vi "Calculate X Y Step Size.vi"(6 "Overlap Options":T3 {"Percent Overlap" max=50}, 7 "Scan Pattern":T1(ring), 8 "Error In":errorcluster, 10 "Y Axis":T2, 11 "X Axis":T2) -> (0 "Error Out":errorcluster, 1 "Array":cluster{"X":dbl, "Y":dbl}[](array[cluster]), 2 "Y Axis Out":T2, 3 "X Axis Out":T2, 4 "size(s)":i32, 5 "# X tiles":i32)   [LabVIEW 2018]
uses:
  Controls/FGV Actions.ctl
panel:
  out "XY Graph":cluster{"X":dbl, "Y":dbl}[](graph)
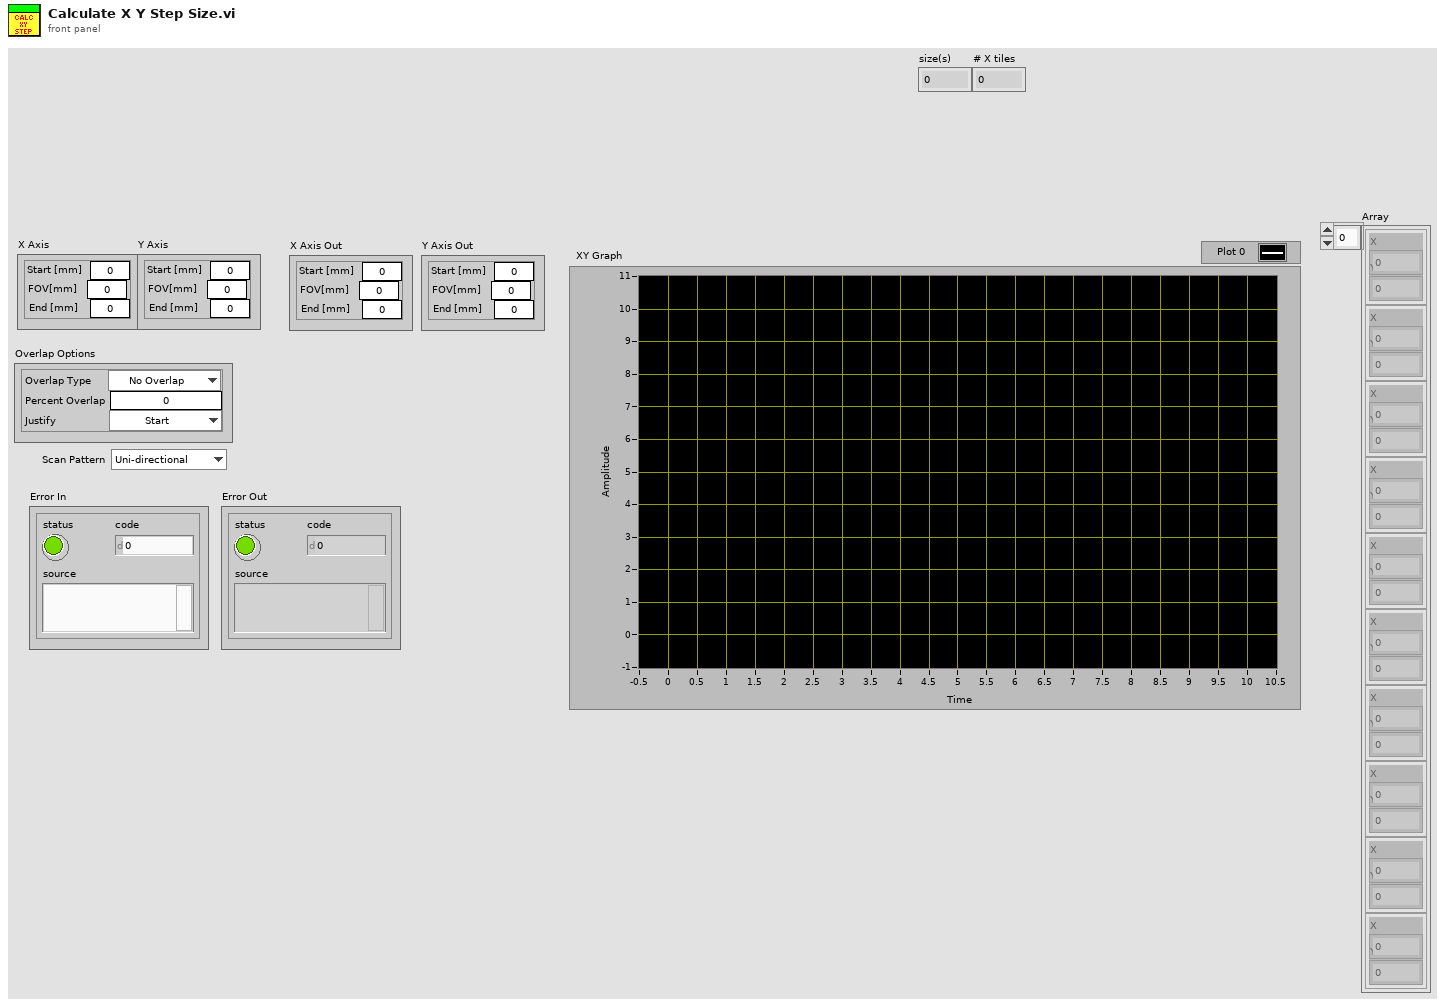
[diagram p1: front panel]
types:
  T1 = enum16{"Uni-directional", "Bi-Directional", "Spiral Out", "Spiral In"}
  T2 = cluster{"Start [mm]":dbl, "FOV[mm]":dbl, "End [mm]":dbl}
  T3 = cluster{"Overlap Type":enum16{"No Overlap", "X Only", "Y Only", "X and Y"}, "Percent Overlap":u8, "Justify":enum16{"Start", "Center", "End"}}
  T4 = typedef "FGV Actions.ctl" = enum16{"Init", "Set", "Get", "Clear"}
  T5 = enum16{"No Overlap", "X Only", "Y Only", "X and Y"}
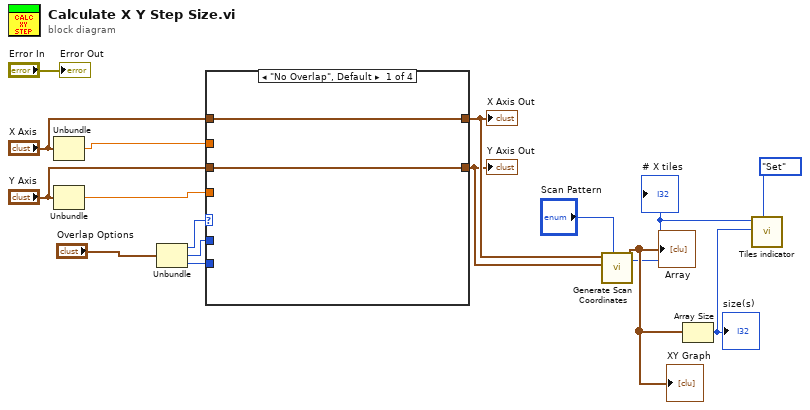
[diagram p0: block diagram]
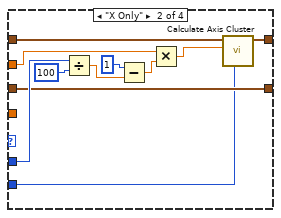
[diagram p2: hidden frame]
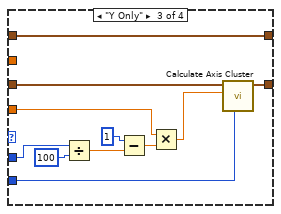
[diagram p3: hidden frame]
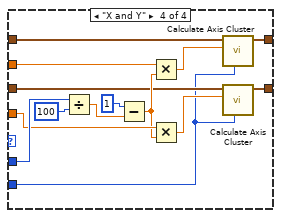
[diagram p4: hidden frame]
diagram:
  n1 = Unbundle("X Axis") -> ("FOV[mm]"=w6:dbl)  [unwired: 2 out]
  n2 = Unbundle("Y Axis") -> ("FOV[mm]"=w5:dbl)  [unwired: 2 out]
  n3 = Unbundle("Overlap Options") -> ("Overlap Type"=w15:T5, "Percent Overlap"=w14:u8, "Justify"=w10:enum16{"Start", "Center", "End"})
  n4 = case shown="\"No Overlap\", Default" w15 {
    tunnel: w14 -> [_ w29 w40 w54]
    tunnel: w5 -> [_ _ w35 w50]
    tunnel: w6 -> [_ w25 _ w48]
    tunnel: "X Axis" -> [w18 w22 w34 w47]
    tunnel: "Y Axis" -> [w17 w23 w32 w46]
    tunnel: [w18 w20 w34 w43] -> w9
    tunnel: [w17 w23 w33 w42] -> w8
    tunnel: w10 -> [_ w19 w30 w41]
    frame "No Overlap", Default {
    }
    frame "X Only" {
      n5 = Divide(x=w29, y=u8 100) -> (x/y=w27:dbl)
      n6 = Subtract(x=u8 1 ("y"), y=w27) -> (x-y=w24:dbl)
      n7 = Multiply(x=w25, y=w24) -> (x*y=w21:dbl)
      n8 = call "Calculate Axis Cluster.vi"("Justify"=w19, "Step Size"=w21, "X Axis in"=w22) -> ("X Axis out"=w20:T2)  [unwired: 8 in]
    }
    frame "Y Only" {
      n9 = Divide(x=w40, y=u8 100) -> (x/y=w38:dbl)
      n10 = Subtract(x=u8 1 ("y"), y=w38) -> (x-y=w36:dbl)
      n11 = Multiply(x=w35, y=w36) -> (x*y=w31:dbl)
      n12 = call "Calculate Axis Cluster.vi"("Justify"=w30, "Step Size"=w31, "X Axis in"=w32) -> ("X Axis out"=w33:T2)  [unwired: 8 in]
    }
    frame "X and Y" {
      n13 = Divide(x=w54, y=u8 100) -> (x/y=w52:dbl)
      n14 = Subtract(x=u8 1 ("y"), y=w52) -> (x-y=w49:dbl)
      n15 = Multiply(x=w48, y=w49) -> (x*y=w45:dbl)
      n16 = Multiply(x=w50, y=w49) -> (x*y=w44:dbl)
      n17 = call "Calculate Axis Cluster.vi"("Justify"=w41, "Step Size"=w45, "X Axis in"=w47) -> ("X Axis out"=w43:T2)  [unwired: 8 in]
      n18 = call "Calculate Axis Cluster.vi"("Justify"=w41, "Step Size"=w44, "X Axis in"=w46) -> ("X Axis out"=w42:T2)  [unwired: 8 in]
    }
  }
  "X Axis Out" <- w9
  "Y Axis Out" <- w8
  n19 = call "Generate Scan Coordinates.vi"("Scan Pattern"="Scan Pattern", "Y Axis"=w8, "X Axis"=w9) -> ("Array"=w4:cluster{"X":dbl, "Y":dbl}[], "# X tiles"=w2:i32)  [unwired: 5 in, 2 out]
  "XY Graph" <- w4
  "Array" <- w4
  "# X tiles" <- w2
  n20 = Array Size(array=w4) -> (size(s)=w1:i32)
  "size(s)" <- w1
  n21 = call "Tiles indicator.vi"("Actions"=FGV_Actions."Set", "# tiles"=w1, "# X tiles"=w2) -> ()  [unwired: 5 in, 4 out]
  "Error Out" <- "Error In"
